vi "CreateEnumClusterTypeDef_all.vi"(5 "BP_Point(0,0)":cluster{"Width":i32, "Height":i32}={"Width"=100, "Height"=36}, 7 "base path":path=path "D:/control", 8 "error in (no error)":errorcluster, 9 "Data":string[][](array[string]), 10 "DataName":string[](array[string]), 11 "VI in":refnum<vi>) -> (0 "error out":errorcluster, 3 "VI out":refnum<vi>)   [LabVIEW 2015]
panel:
  out "Cluster out":refnum<vi>
  in  "FP_Point(0,0)":cluster{"Width":i32, "Height":i32}={"Width"=100, "Height"=36}
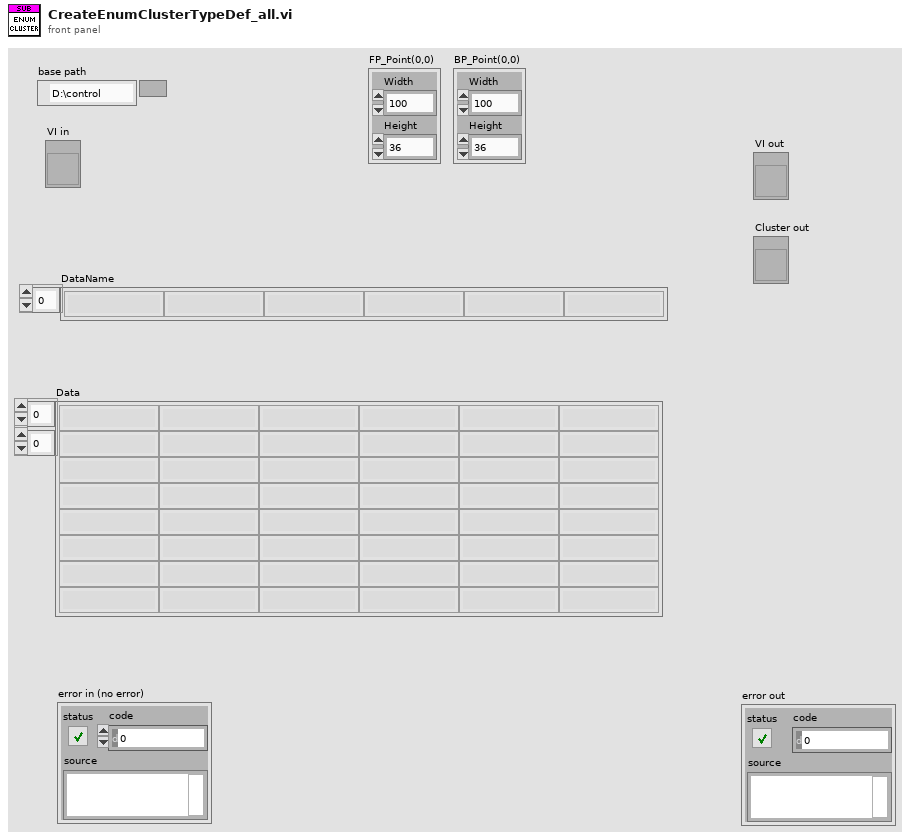
[diagram p1: front panel]
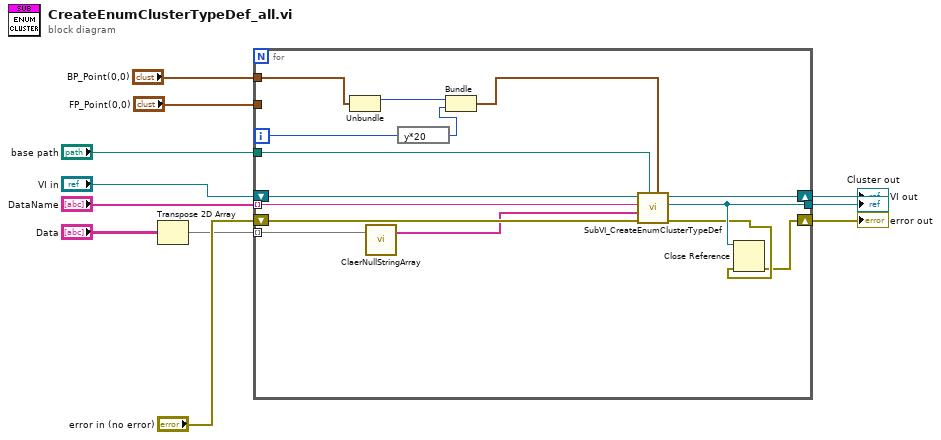
[diagram p0: block diagram]
diagram:
  n1 = Transpose 2D Array(2D array="Data") -> (transposed array=w4:string[][])
  n2 = for {
    tunnel: "BP_Point(0,0)" -> [w19]
    tunnel: "FP_Point(0,0)" -> [_]
    tunnel: w4 -> [w16] mode=indexing
    tunnel: "DataName" -> [w24] mode=indexing
    tunnel: [w14] -> w6
    shift-right: [w23] -> w5
    shift-left: "VI in" -> [w26]
    shift-right: [w12] -> w7
    shift-left: "error in (no error)" -> [w25]
    tunnel: "base path" -> [w17]
    i -> [w20]
    n3 = Unbundle(w19) -> ("Width"=w22:i32)  [unwired: 1 out]
    n4 = call <userlib>:"ClaerNullStringArray.vi"("Array in"=w16) -> ("Array out"=w15:string[])  [unwired: 18 in]
    n5 = expression code="y*20"(w20) -> (w21:i32)
    n6 = Bundle("Width"=w22, w21) -> (w18:cluster{"Width":i32, i32})  [unwired: 1 in]
    n7 = call "SubVI_CreateEnumClusterTypeDef.vi"("BP_Point(0,0)"=w18, "base path"=w17, "error in (no error)"=w25, "Data"=w15, "Name"=w24, "VI in"=w26) -> ("error out"=w13:errorcluster, "Cluster out"=w14:refnum<vi>, "VI out"=w23:refnum<vi>)  [unwired: 3 in]
    n8 = Close Reference(reference=w14, error in (no error)=w13) -> (error out=w12:errorcluster)
  }
  "error out" <- w7
  "Cluster out" <- w6
  "VI out" <- w5
